vi "SPI Engine. Send SPI Device Response Data.vi"(8 "error in":errorcluster, 9 "Input Valid":bool, 10 "Input Data":T1, 11 "Private Data In":T2={"DLU To SPI Engine Data FIFO"="DLU To SPI Engine Data", "SPI Engine to DLU Data FIFO"="SPI Engine to DLU Data", "Data to SPI Engine (Cache) Register"="Data to SPI Engine (Cache)", "SPI PHY Settings to SPI Engine (Cahche) Register"="SPI PHY Settings to SPI Engine (Cache)"}) -> (0 "error out":errorcluster, 1 "New Data Sent?":bool, 2 "Output Data":T1, 4 "Ready for Input":bool)   [LabVIEW 2014]
doc: "This VI conditionally writes new data to the SPI Response FIFO."
uses:
  Controls/SPI Response Information.ctl
  Controls/Internal Data (SPI API).ctl
panel:
  out "Data Sent_First":T1
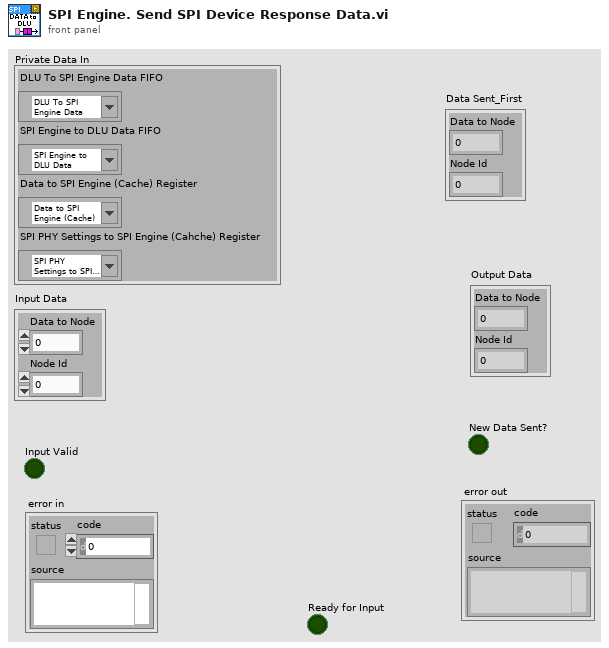
[diagram p1: front panel]
types:
  T1 = typedef "SPI Response Information.ctl" = cluster{"Data to Node":u64, "Node Id":u16}
  T2 = typedef "Internal Data (SPI API).ctl" = cluster{"DLU To SPI Engine Data FIFO":refnum<k21>, "SPI Engine to DLU Data FIFO":refnum<k21>, "Data to SPI Engine (Cache) Register":refnum<k21>, "SPI PHY Settings to SPI Engine (Cahche) Register":refnum<k21>}
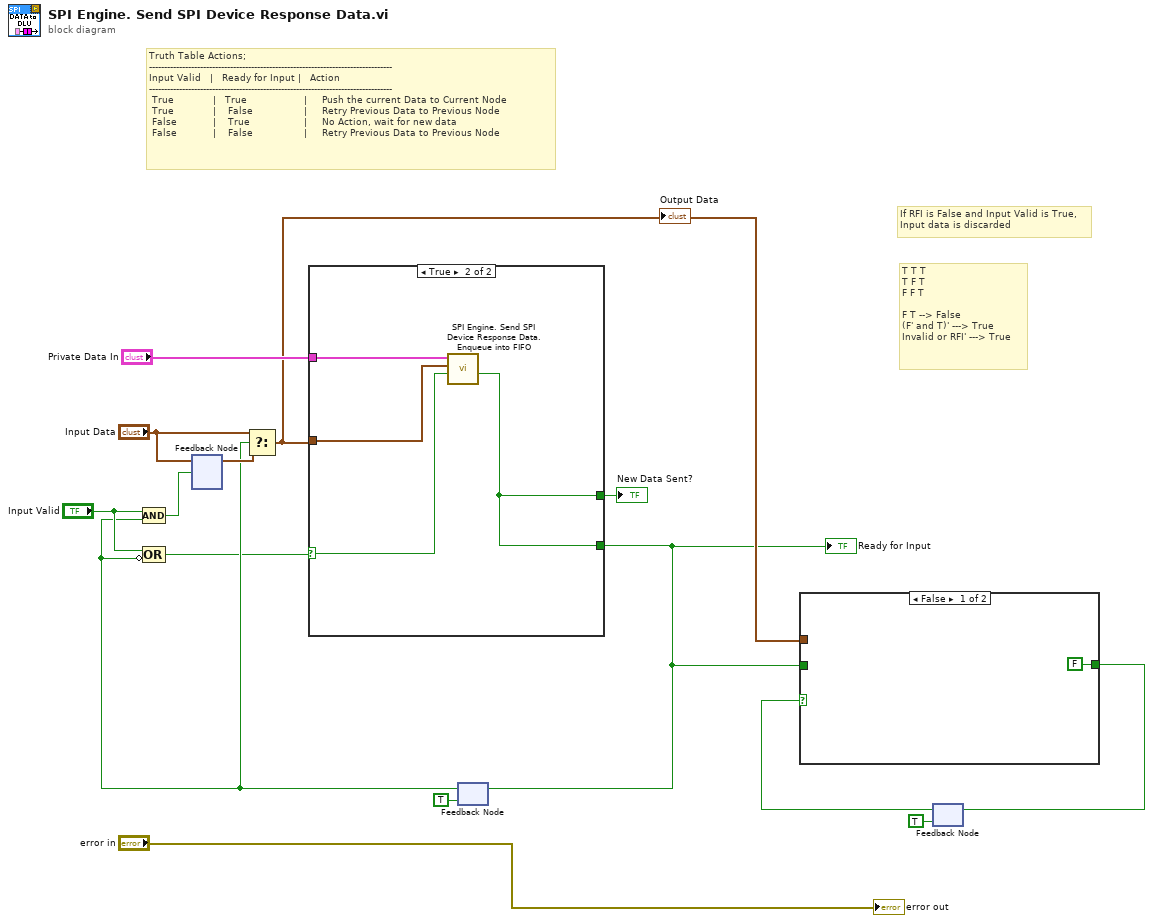
[diagram p0: block diagram]
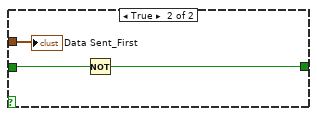
[diagram p2: hidden frame]
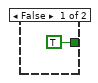
[diagram p3: hidden frame]
diagram:
  # "T T T\nT F T\nF F T\n\nF T --> False\n(F' and T)' ---> True\nInvalid or RFI' ---> True"
  # "If RFI is False and Input Valid is True,\nInput data is discarded"
  # "Truth Table Actions;\n---------------------------------------------------------------------------------\nInput Valid   |   Ready for Input |   Action\n---------------------------------------------------------------------------------\n True             |   True                   |     Push the current Data to Current Node\n True             |    False                 |     Retry Previous Data to Previous Node\n False            |    True                  |     No Action, wait for new data\n False            |    False                 |     Retry Previous Data to Previous Node"
  n1 = feedback #1() -> (w12:T1)  [unwired: 1 in]
  n2 = feedback #2(TRUE ("Send Success?")) -> (w7:bool)
  n3 = Compound Arithmetic op=AND("Input Valid", w7) -> (w14:bool)
  n4 = Compound Arithmetic op=OR("Input Valid", invert w7) -> (w6:bool)
  n5 = feedback-in #1("Input Data", w14) -> ()
  n6 = Select(t="Input Data", s=w7, f=w12) -> (s? t:f=w5:T1)
  "Output Data" <- w5
  n7 = case shown="True" w6 {
    selector: w6 -> [_ w18]
    tunnel: "Private Data In" -> [_ w20]
    tunnel: w5 -> [_ w19]
    tunnel: [TRUE ("Send Success?") w17] -> w4
    tunnel: [_ w17] -> w8
    frame False {
    }
    frame True {
      n8 = call "SPI Engine. Send SPI Device Response Data. Enqueue into FIFO.vi"("Input Valid"=w18, "Input Data"=w19, "Private Data In"=w20) -> ("Send Success?"=w17:bool)  [unwired: 7 in, 1 out]
    }
  }
  "Ready for Input" <- w4
  "New Data Sent?" <- w8
  n9 = feedback-in #2(w4) -> ()
  n10 = feedback #3(TRUE) -> (w2:bool)
  n11 = case shown="False" w2 {
    tunnel: w5 -> [_ w24]
    tunnel: w4 -> [_ w23]
    tunnel: [FALSE w22] -> w3
    frame False {
    }
    frame True {
      n12 = Not(x=w23) -> (.not. x?=w22:bool)
      "Data Sent_First" <- w24
    }
  }
  n13 = feedback-in #3(w3) -> ()
  "error out" <- "error in"
